vi "Create Animation.vi"(2 "L/R":bool, 4 "Target Values":T3={"Target Shouler Angle"=120.0, "Target Shoulder Axis"={"X"=-1.0, "Y"=0.0, "Z"=0.0}, "Target Elbow Angle"=0.0, "Target Elbow Axis"={"X"=0.0, "Y"=-1.0, "Z"=0.0}, "Humerus rel Trunk"=[], "AP Translation"={"X"=0.0, "Y"=-1.0, "Z"=0.0}}) -> (0 "Arm Refs":T1, 1 "Scene Out":refnum<vi>)   [LabVIEW 2010]
uses:
  <vilib>/Analysis/Matrix/Datatypes/RealMatrix.ctl
  <vilib>/picture/3D Picture Control/NI_3D Picture Control.lvlib
  <vilib>/Analysis/Matrix/NI_Matrix.lvlib
panel:
  out "AP Translation":cluster{"X":dbl, "Y":dbl, "Z":dbl}
  out "L SJC":refnum<vi>
  out "R SJC":refnum<vi>
  out "R Arm":refnum<vi>
  out "Target Elbow Axis":cluster{"X":dbl, "Y":dbl, "Z":dbl}
  out "Target Elbow Angle":dbl
  out "Target Shoulder Axis":cluster{"X":dbl, "Y":dbl, "Z":dbl}
  out "Target Shouler Angle":dbl
  out "L EJC":refnum<vi>
  out "L Arm":refnum<vi>
  out "R EJC":refnum<vi>
  # "Left"
  # "Right"
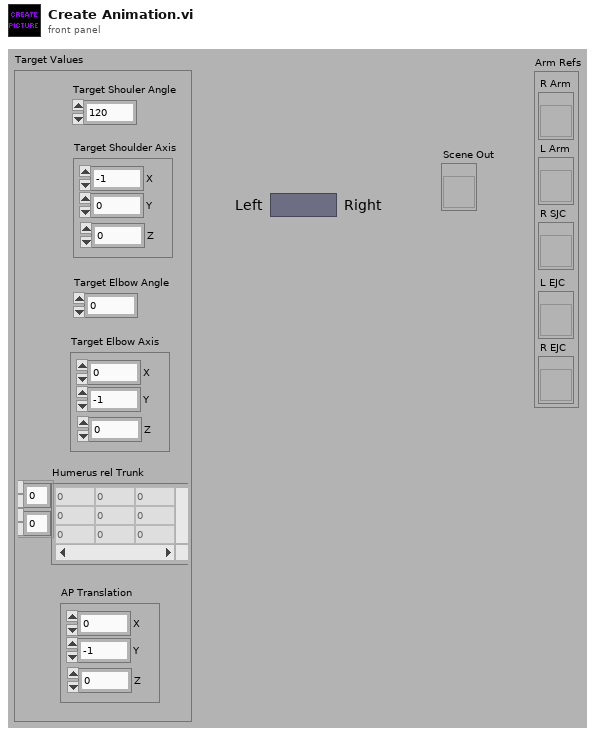
[diagram p1: front panel]
types:
  T1 = cluster{"R Arm":refnum<vi>, "L Arm":refnum<vi>, "R SJC":refnum<vi>, "L EJC":refnum<vi>, "R EJC":refnum<vi>}
  T2 = typedef "NI_Matrix.lvlib/RealMatrix.ctl" = dbl[][]
  T3 = cluster{"Target Shouler Angle":dbl, "Target Shoulder Axis":cluster{"X":dbl, "Y":dbl, "Z":dbl}, "Target Elbow Angle":dbl, "Target Elbow Axis":cluster{"X":dbl, "Y":dbl, "Z":dbl}, "Humerus rel Trunk":T2, "AP Translation":cluster{"X":dbl, "Y":dbl, "Z":dbl}}
  T4 = cluster{"Radius":sgl, "Name":string, "Height":sgl, "Radius":sgl, "RGBA":cluster{"R":sgl, "G":sgl, "B":sgl, "A":sgl}}
  T5 = cluster{"reference out":refnum<vi>, "Name":string, "Height":sgl, "Radius":sgl}
  T6 = cluster{"R SJC":refnum<vi>, "R EJC":refnum<vi>, dbl, cluster{"X":dbl, "Y":dbl, "Z":dbl}, dbl, cluster{"X":dbl, "Y":dbl, "Z":dbl}}
  T7 = cluster{"Axis":cluster{"X":sgl, "Y":sgl, "Z":sgl}, "L Arm":refnum<vi>, "L EJC":refnum<vi>, dbl, cluster{dbl, "Y":dbl, "Z":dbl}, dbl, cluster{"X":dbl, "Y":dbl, "Z":dbl}}
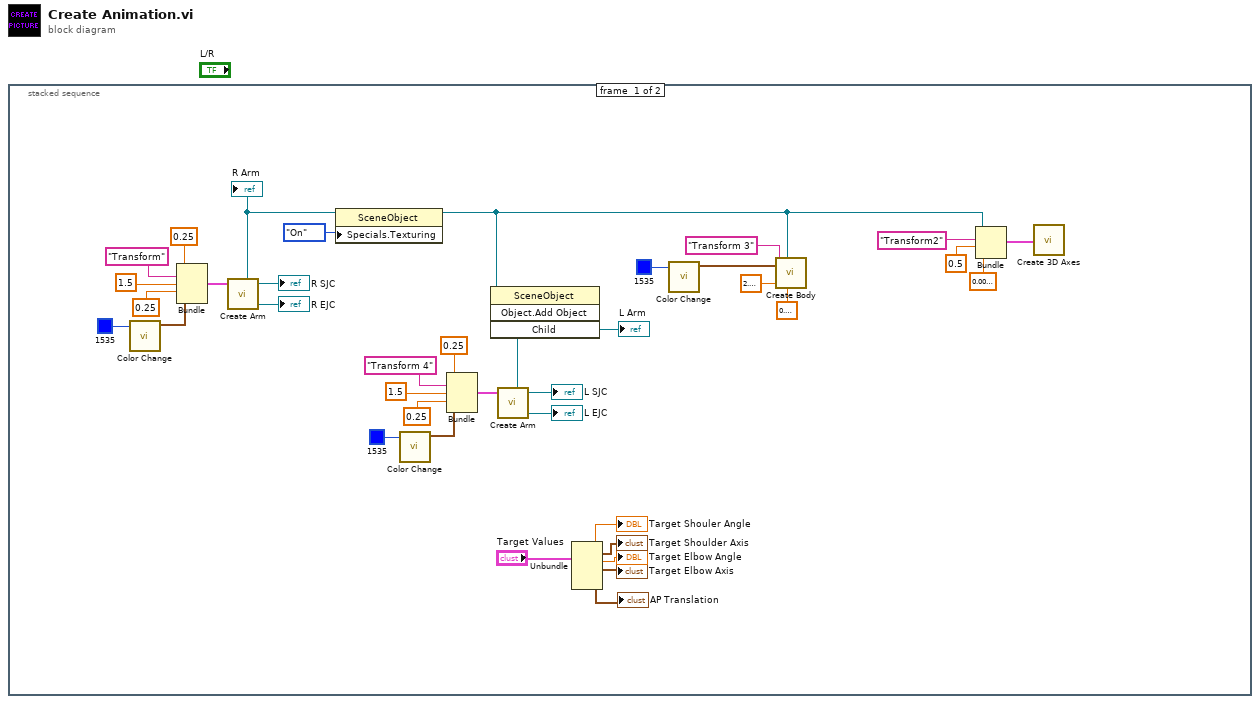
[diagram p0: block diagram]
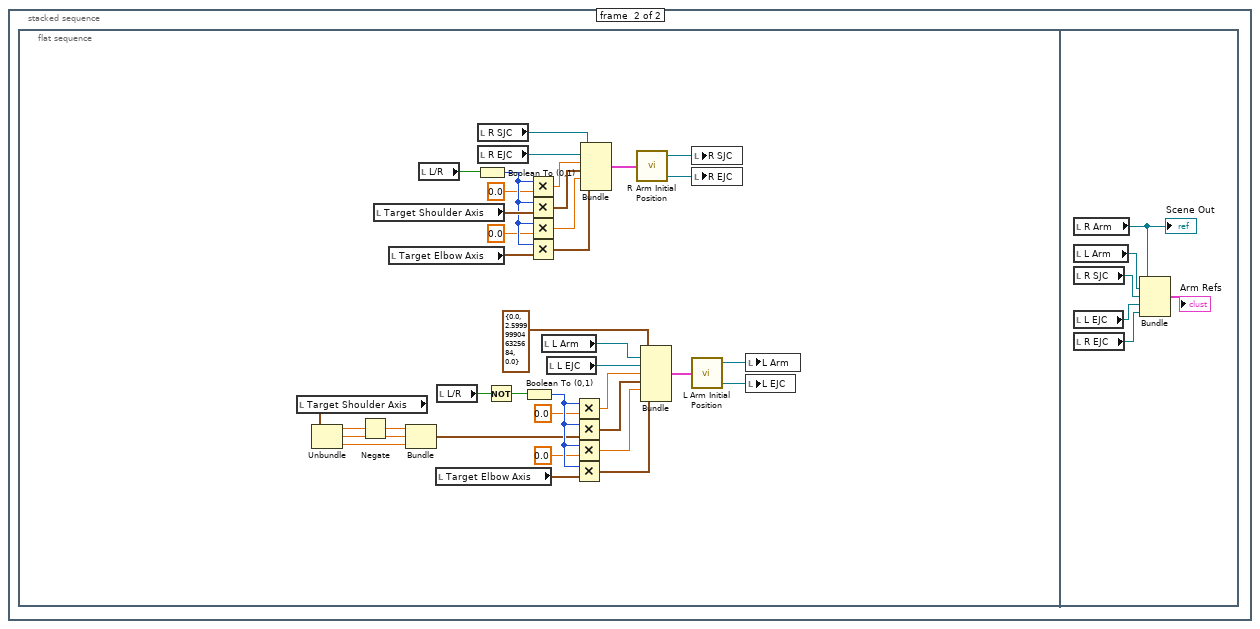
[diagram p2: hidden frame]
diagram:
  n1 = stacked-sequence {
    frame #0 {
      n2 = call <vilib>:"Color Change.vi"("Color"=u32 1535) -> ("RGBA"=w22:cluster{"R":sgl, "G":sgl, "B":sgl, "A":sgl})  [unwired: 10 in]
      n3 = Bundle("Radius"=sgl 0.25, "Name"="Transform", "Height"=sgl 1.5, "Radius"=sgl 0.25, "RGBA"=w22) -> (w21:T4)  [unwired: 1 in]
      n4 = call "Create Arm.vi"("Arm Cluster"=w21) -> ("EJC"=→"R EJC":refnum<vi>, "SJC"=→"R SJC":refnum<vi>, "reference out"=w20:refnum<vi>)  [unwired: 3 in, 1 out]
      "R Arm" <- w20
      n5 = property class="SceneObject"(reference=w20, "Specials.Texturing"=enum16{"Inherit Value", "Off", "On"}."On" ("Specials:Texturing")) -> (reference out=w26:refnum<vi>)  [unwired: 1 in, 1 out]
      n6 = call <vilib>:"Color Change.vi"("Color"=u32 1535) -> ("RGBA"=w30:cluster{"R":sgl, "G":sgl, "B":sgl, "A":sgl})  [unwired: 10 in]
      n7 = Bundle("Radius"=sgl 0.25, "Name"="Transform 4", "Height"=sgl 1.5, "Radius"=sgl 0.25, "RGBA"=w30) -> (w18:T4)  [unwired: 1 in]
      n8 = call "Create Arm.vi"("Arm Cluster"=w18) -> ("EJC"=→"L EJC":refnum<vi>, "SJC"=→"L SJC":refnum<vi>, "reference out"=w16:refnum<vi>)  [unwired: 3 in, 1 out]
      n9 = invoke class="SceneObject" method="Object.Add Object"(reference=w26, "Child"=w16) -> ("Child"=→"L Arm":refnum<vi>)  [unwired: 2 in, 3 out]
      n10 = Unbundle("Target Values") -> ("Target Shouler Angle"=→"Target Shouler Angle":dbl, "Target Shoulder Axis"=→"Target Shoulder Axis":cluster{"X":dbl, "Y":dbl, "Z":dbl}, "Target Elbow Angle"=→"Target Elbow Angle":dbl, "Target Elbow Axis"=→"Target Elbow Axis":cluster{"X":dbl, "Y":dbl, "Z":dbl}, "AP Translation"=→"AP Translation":cluster{"X":dbl, "Y":dbl, "Z":dbl})  [unwired: 1 out]
      n11 = call <vilib>:"Color Change.vi"("Color"=u32 1535) -> ("RGBA"=w23:cluster{"R":sgl, "G":sgl, "B":sgl, "A":sgl})  [unwired: 10 in]
      n12 = call "Create Body.vi"("Name"="Transform 3", "Origin"=w26, "Color"=w23, "Height"=sgl 2.3, "Radius"=sgl 0.7) -> ()  [unwired: 2 in, 2 out]
      n13 = Bundle("reference out"=w26, "Name"="Transform2", "Height"=sgl 0.5, "Radius"=sgl 0.01) -> (w12:T5)  [unwired: 1 in]
      n14 = call "Create 3D Axes.vi"("Cluster"=w12) -> ()  [unwired: 1 in]
    }
    frame #1 {
      n15 = flat-sequence {
        frame #0 {
          n16 = local read "Target Shoulder Axis"() -> (w43:cluster{"X":dbl, "Y":dbl, "Z":dbl})
          n17 = Unbundle(w43) -> ("X"=w49:dbl, "Y"=w47:dbl, "Z"=w46:dbl)
          n18 = Negate(x=w49) -> (-x=w48:dbl)
          n19 = local read "Target Shoulder Axis"() -> (w71:cluster{"X":dbl, "Y":dbl, "Z":dbl})
          n20 = local read "Target Elbow Axis"() -> (w69:cluster{"X":dbl, "Y":dbl, "Z":dbl})
          n21 = Bundle(w48, "Y"=w47, "Z"=w46) -> (w44:cluster{dbl, "Y":dbl, "Z":dbl})  [unwired: 1 in]
          n22 = local read "L/R"() -> (w63:bool)
          n23 = local read "Target Elbow Axis"() -> (w53:cluster{"X":dbl, "Y":dbl, "Z":dbl})
          n24 = local read "L/R"() -> (w57:bool)
          n25 = Boolean To (0,1)(Boolean=w63) -> (0, 1=w64:i16)
          n26 = local read "R SJC"() -> (w73:refnum<vi>)
          n27 = local read "R EJC"() -> (w70:refnum<vi>)
          n28 = Not(x=w57) -> (.not. x?=w56:bool)
          n29 = Boolean To (0,1)(Boolean=w56) -> (0, 1=w62:i16)
          n30 = Multiply(x=w64, y=0.0) -> (x*y=w65:dbl)
          n31 = Multiply(x=w64, y=w71) -> (x*y=w66:cluster{"X":dbl, "Y":dbl, "Z":dbl})
          n32 = Multiply(x=w64, y=0.0) -> (x*y=w67:dbl)
          n33 = Multiply(x=w64, y=w69) -> (x*y=w68:cluster{"X":dbl, "Y":dbl, "Z":dbl})
          n34 = local read "L Arm"() -> (w54:refnum<vi>)
          n35 = local read "L EJC"() -> (w61:refnum<vi>)
          n36 = Multiply(x=w62, y=0.0) -> (x*y=w60:dbl)
          n37 = Multiply(x=w62, y=w44) -> (x*y=w45:cluster{dbl, "Y":dbl, "Z":dbl})
          n38 = Multiply(x=w62, y=0.0) -> (x*y=w59:dbl)
          n39 = Multiply(x=w62, y=w53) -> (x*y=w58:cluster{"X":dbl, "Y":dbl, "Z":dbl})
          n40 = Bundle("R SJC"=w73, "R EJC"=w70, w65, w66, w67, w68) -> (w72:T6)  [unwired: 1 in]
          n41 = call "R Arm Initial Position.vi"("Cluster"=w72) -> ("Scene.Object Out"=w75:refnum<vi>, "Scene.Object Out 3"=w74:refnum<vi>)  [unwired: 1 in]
          n42 = Bundle("Axis"=cluster{"X":sgl, "Y":sgl, "Z":sgl} {"X"=0.0, "Y"=2.6, "Z"=0.0}, "L Arm"=w54, "L EJC"=w61, w60, w45, w59, w58) -> (w52:T7)  [unwired: 1 in]
          n43 = local write "R SJC"(w74) -> ()
          n44 = local write "R EJC"(w75) -> ()
          n45 = call "L Arm Initial Position.vi"("Cluster"=w52) -> ("Scene.Object Out"=w50:refnum<vi>, "Scene.Object Out 3"=w51:refnum<vi>)  [unwired: 1 in]
          n46 = local write "L Arm"(w51) -> ()
          n47 = local write "L EJC"(w50) -> ()
        }
        frame #1 {
          n48 = local read "R Arm"() -> (w77:refnum<vi>)
          "Scene Out" <- w77
          n49 = local read "L Arm"() -> (w78:refnum<vi>)
          n50 = local read "R SJC"() -> (w79:refnum<vi>)
          n51 = local read "L EJC"() -> (w81:refnum<vi>)
          n52 = local read "R EJC"() -> (w80:refnum<vi>)
          n53 = Bundle("R Arm"=w77, "L Arm"=w78, "R SJC"=w79, "L EJC"=w81, "R EJC"=w80) -> (→"Arm Refs":T1)  [unwired: 1 in]
        }
      }
    }
  }
